vi "ConfigurePower.vi"(8 "error in (no error)":errorcluster, 9 "Port":i32 caption="PortVal" format="%.0g", 10 "Power Level":dbl=-20.0 format="%#_13g", 11 "NetA_AgNA in":refnum<class "NetA_AgNA.lvclass">) -> (0 "error out":errorcluster, 3 "NetA_AgNA out":refnum<class "NetA_AgNA.lvclass">)   [LabVIEW 2014, in "NetA_AgNA.lvclass"]
doc: "Configure power level. Alternative to the Agilent NA.lvlib (did not understand how to use port value)."
uses:
  NetA_AgNA.lvclass
  NetA_AgNA.lvclass/NetA_AgNA.ctl
  data/Agilent NA.lvlib
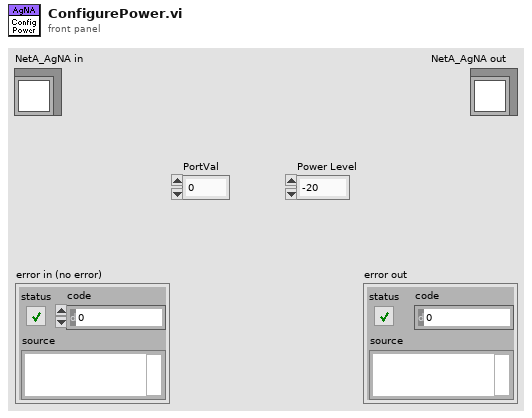
[diagram p1: front panel]
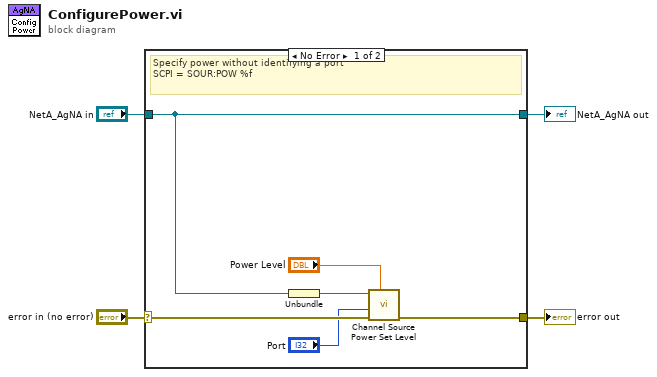
[diagram p0: block diagram]
diagram:
  n1 = case shown="No Error" "error in (no error)" {
    selector: "error in (no error)" -> [w9 w12]
    tunnel: [w7 w12] -> w3
    tunnel: "NetA_AgNA in" -> [w10 w11]
    tunnel: [w10 w11] -> w1
    frame No Error {
      # "Specify power without identifying a port\nSCPI = SOUR:POW %f"
      n2 = Unbundle(w10) -> (w8:refnum<k15>)
      n3 = call "Channel Source Power Set Level.vi"("Val"="Power Level", "error in (no error)"=w9, "PortVal"="Port", "instrument handle"=w8) -> ("error out"=w7:errorcluster)  [unwired: 6 in, 1 out]
    }
    frame Error {
    }
  }
  "error out" <- w3
  "NetA_AgNA out" <- w1
